vi "Bind RPC getCANDatafromrgrpcServer_clientRequester_getIDFormServer.vi"(11 "gRPCid server in":T3) -> (0 "error out":errorcluster, 1 "getCANDatafromrgrpcServer_clientRequester_getIDFormServer Internal UE":T2, 2 "getCANDatafromrgrpcServer_clientRequester_getIDFormServer gRPC UE":T1, 3 "gRPCid server out":T3)   [LabVIEW 2020, in "server1.lvlib" / "server1.lvclass"]
uses:
  server1.lvclass
  gRPC lvSupport/Server API/typeDefs/grpcId.ctl
  typeDefs/Server Internal Message UE.ctl
  typeDefs/Server Internal Message.ctl
  gRPC lvSupport/Server API/typeDefs/gRPCId Cluster UE.ctl
  gRPC lvSupport/Server API/typeDefs/gRPCId Cluster.ctl
  616620f9-6bbe-466a-af51-04bcc3596ea0.vi
  gRPC lvSupport/Server API/Server/Get Server DLL Path.vi
  server1.lvclass/server1.ctl
  gRPC lvSupport/gprc-lvsupport.lvlib
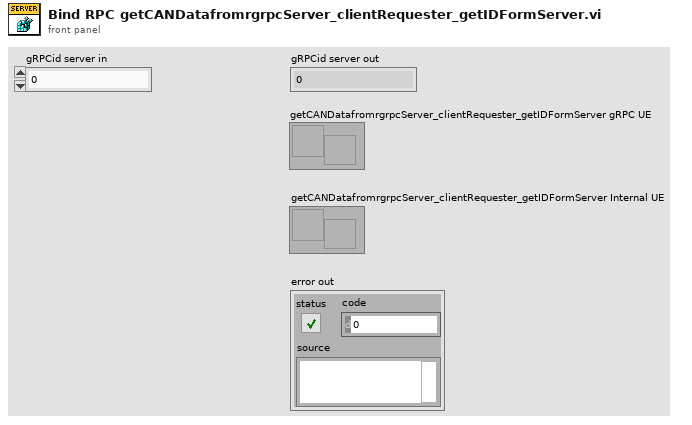
[diagram p1: front panel]
types:
  T1 = typedef "server1.lvlib/gprc-lvsupport.lvlib/gRPCId Cluster UE.ctl" = refnum<user-event>
  T2 = typedef "server1.lvlib/server1.lvclass/Server Internal Message UE.ctl" = refnum<user-event>
  T3 = typedef "server1.lvlib/gprc-lvsupport.lvlib/grpcId.ctl" = u64
  T4 = typedef "server1.lvlib/server1.lvclass/Server Internal Message.ctl" = cluster{"Command":string, "Data":variant}
  T5 = typedef "server1.lvlib/gprc-lvsupport.lvlib/gRPCId Cluster.ctl" = cluster{"gRPCid":T3}
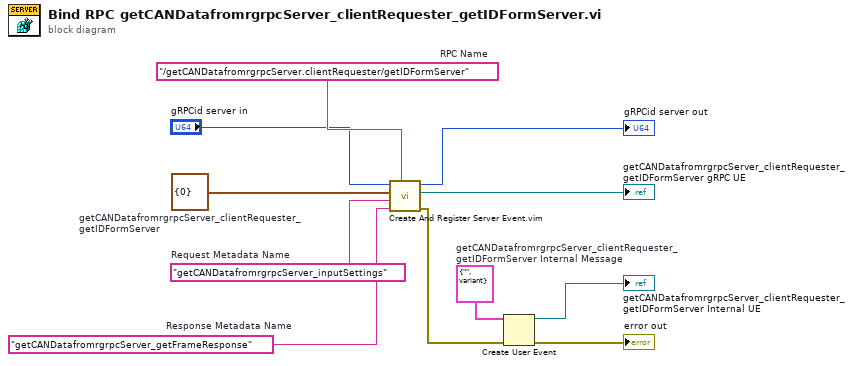
[diagram p0: block diagram]
diagram:
  w5 = T4 {"Command"="", "Data"=variant}  # getCANDatafromrgrpcServer_clientRequester_getIDFormServer Internal Message
  w8 = "getCANDatafromrgrpcServer_getFrameResponse"  # Response Metadata Name
  w11 = T5 {"gRPCid"=0}  # getCANDatafromrgrpcServer_clientRequester_getIDFormServer
  w9 = "getCANDatafromrgrpcServer_inputSettings"  # Request Metadata Name
  w10 = "/getCANDatafromrgrpcServer.clientRequester/getIDFormServer"  # RPC Name
  n1 = call "Create And Register Server Event.vim"("Method name"=w10, "Response Metadata Name"=w8, "Request Metadata Name"=w9, "event in"=w11, "gRPCid server in"="gRPCid server in") -> ("error out"=w4:errorcluster, "event"=→"getCANDatafromrgrpcServer_clientRequester_getIDFormServer gRPC UE":refnum<user-event>, "gRPCid server out"=→"gRPCid server out":T3)  [unwired: 4 in]
  n2 = Create User Event(user event datatype=w5, error in=w4) -> (user event=→"getCANDatafromrgrpcServer_clientRequester_getIDFormServer Internal UE":refnum<user-event>, error out=→"error out":errorcluster)
